vi "Configure Trigger (Video).vi"(0 "VISA resource name":refnum<visa-resource-name>, 1 "Polarity (1: Positive)":u16(ring)=1 items=["Negative", "Positive", "Normal", "Inverted"], 2 "Holdoff Fields (0)":dbl, 5 "Trigger Source (0: Channel 1)":u16(ring) items=["Channel 1"=0, "Channel 2"=1, "Channel 3"=2, "Channel 4"=3, "Digital Channel 0"=14, "Digital Channel 1"=15, "Digital Channel 2"=16, "Digital Channel 3"=17, "Digital Channel 4"=18, "Digital Channel 5"=19, "Digital Channel 6"=20, "Digital Channel 7"=21, "Digital Channel 8"=22, "Digital Channel 9"=23, "Digital Channel 10"=24, "Digital Channel 11"=25, "Digital Channel 12"=26, "Digital Channel 13"=27, "Digital Channel 14"=28, "Digital Channel 15"=29], 7 "Signal Format (0: NTSC)":u16(ring) items=["NTSC", "PAL", "SECAM", "HDTV"], 9 "Trigger Event (0: Odd Fields)":u16(ring) items=["Odd Fields", "Even Fields", "All Fields", "All Lines", "Numeric"], 11 "error in (no error)":errorcluster, 12 "HDTV Format (0: HD1080P24)":u16(ring) items=["HD1080P24", "HD720P60", "HD480P60", "HD1080I50", "HD1080P25", "HD1080I60", "HD1080PSF24", "HD576P50", "HD720P30", "HD720P50", "HD875I60", "HD1080P30", "HD1080P50", "HD1080P60"], 13 "Video Trigger Line (1)":dbl=1.0) -> (4 "VISA resource name out":refnum<visa-resource-name>, 15 "error out":errorcluster)   [LabVIEW 2009, in "Tektronix DPO MSO 2000 4000 Series.lvlib"]
doc: "Configures video trigger settings for an oscilloscope."
uses:
  <instrlib>/Tektronix DPO MSO 2000 4000 Series/Tektronix DPO MSO 2000 4000 Series.lvlib
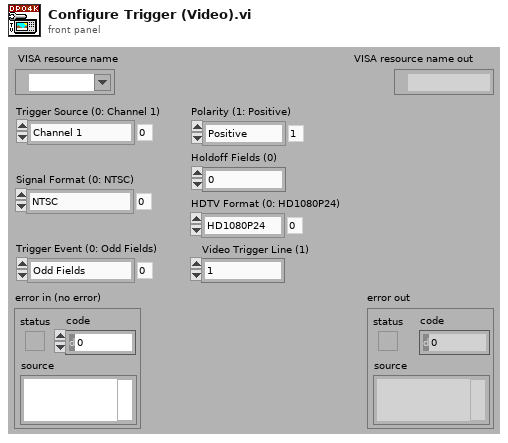
[diagram p1: front panel]
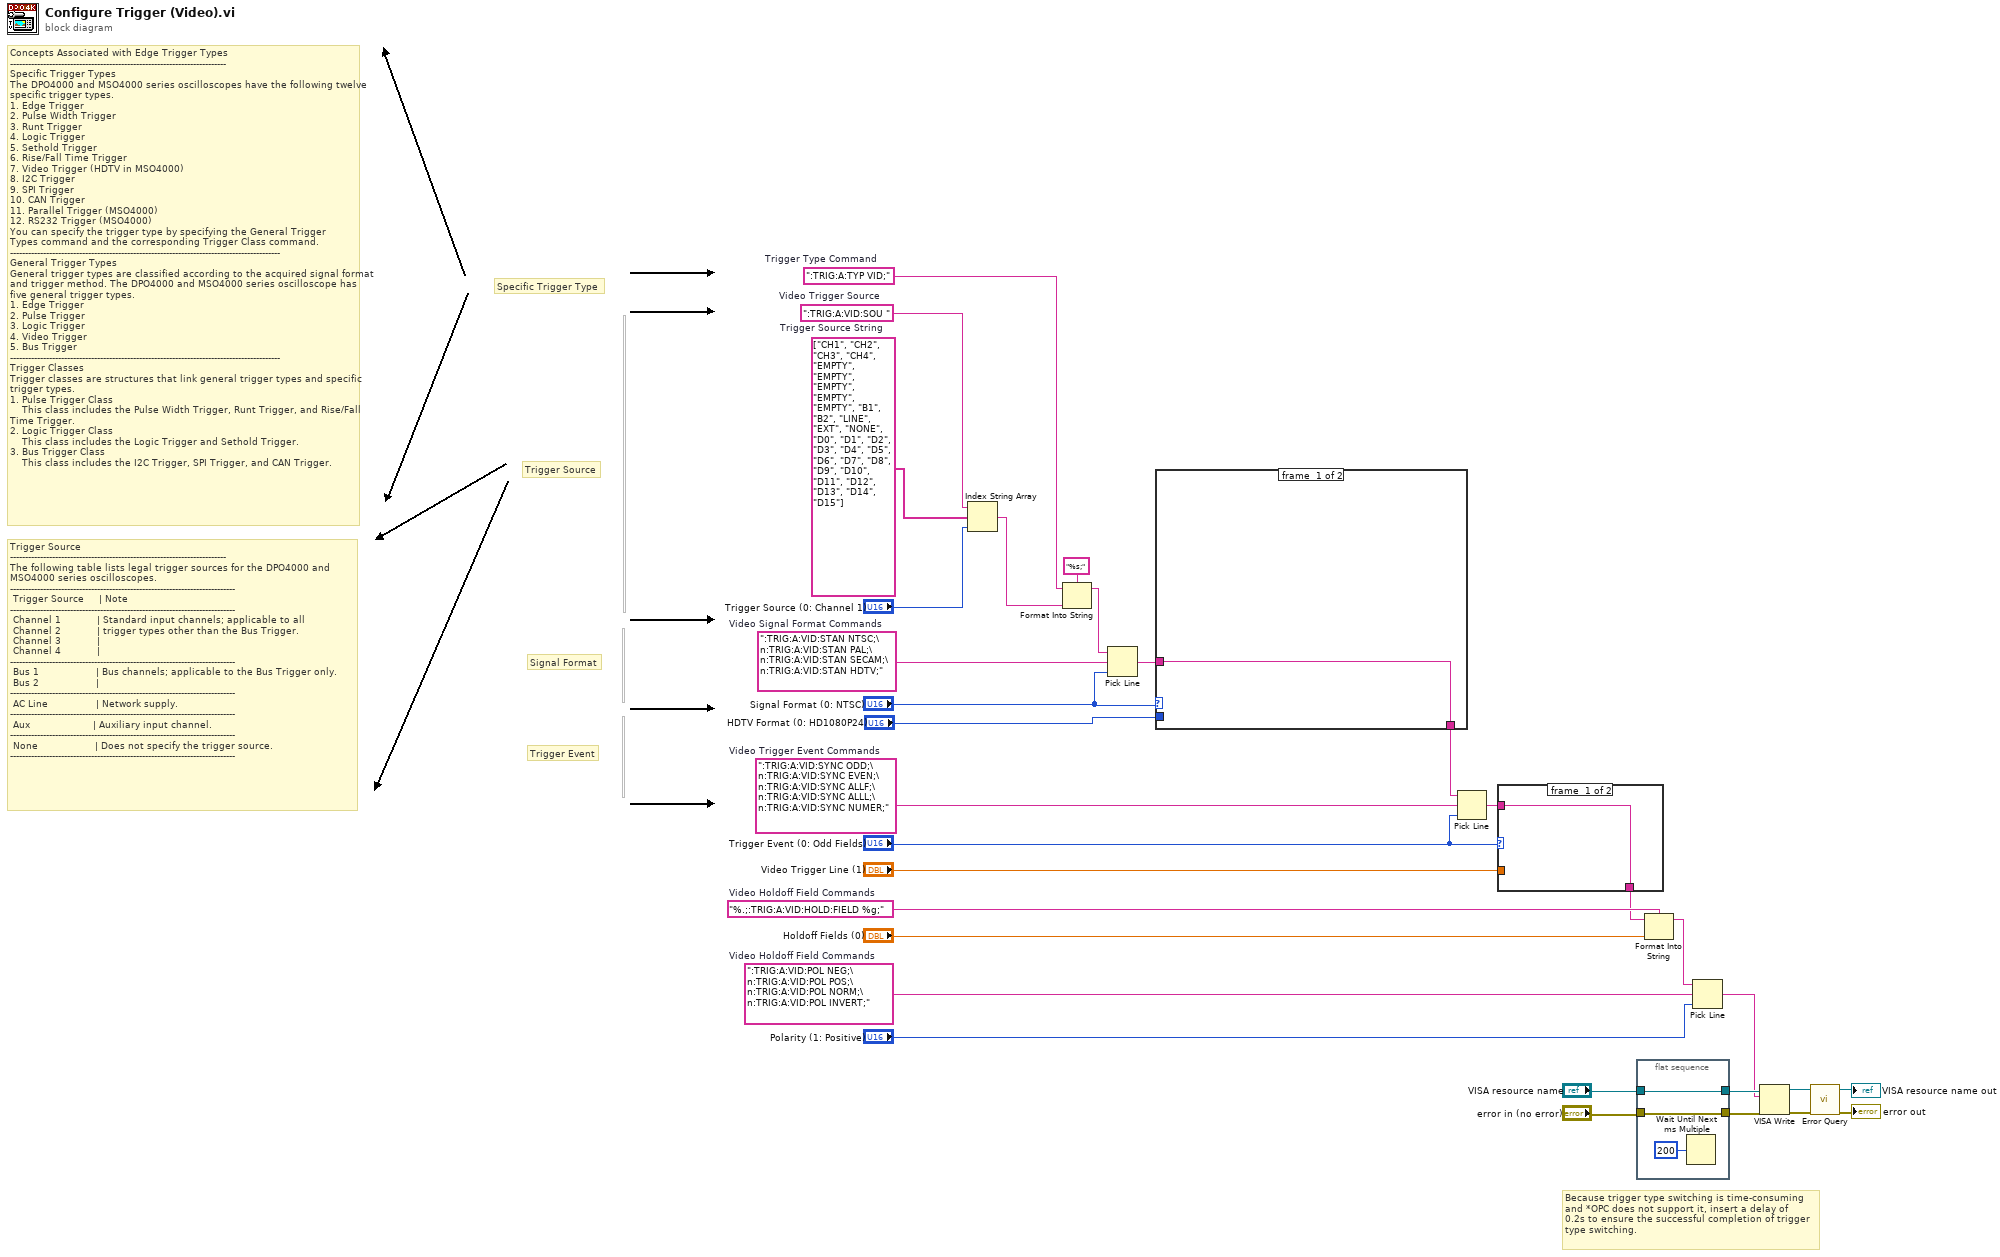
[diagram p0: block diagram]
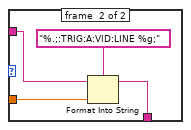
[diagram p2: hidden frame]
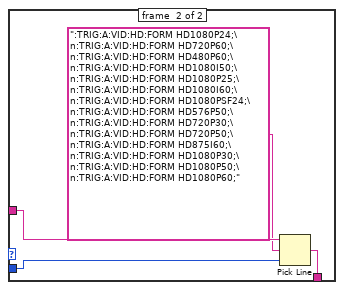
[diagram p3: hidden frame]
diagram:
  w3 = ":TRIG:A:VID:POL NEG;\n:TRIG:A:VID:POL POS;\n:TRIG:A:VID:POL NORM;\n:TRIG:A:VID:POL INVERT;"  # Video Holdoff Field Commands
  w7 = "%.;:TRIG:A:VID:HOLD:FIELD %g;"  # Video Holdoff Field Commands
  w19 = ":TRIG:A:TYP VID;"  # Trigger Type Command
  w20 = string[] ["CH1", "CH2", "CH3", "CH4", "EMPTY", "EMPTY", "EMPTY", "EMPTY", "EMPTY", "B1", "B2", "LINE", "EXT", "NONE", "D0", "D1", "D2", "D3", "D4", "D5", "D6", "D7", "D8", "D9", "D10", "D11", "D12", "D13", "D14", "D15"]  # Trigger Source String
  w22 = ":TRIG:A:VID:SYNC ODD;\n:TRIG:A:VID:SYNC EVEN;\n:TRIG:A:VID:SYNC ALLF;\n:TRIG:A:VID:SYNC ALLL;\n:TRIG:A:VID:SYNC NUMER;"  # Video Trigger Event Commands
  w24 = ":TRIG:A:VID:STAN NTSC;\n:TRIG:A:VID:STAN PAL;\n:TRIG:A:VID:STAN SECAM;\n:TRIG:A:VID:STAN HDTV;"  # Video Signal Format Commands
  w30 = ":TRIG:A:VID:SOU "  # Video Trigger Source
  # "Trigger Source\n------------------------------------------------------------------------\nThe following table lists legal trigger sources for the DPO4000 and MSO4000 series oscilloscopes.\n---------------------------------------------------------------------------\n Trigger Source     | Note                                                           \n---------------------------------------------------------------------------\n Channel 1            | Standard input channels; applicable to all      \n Channel 2            | trigger types other than the Bus Trigger.         \n Channel 3            |     \n Channel 4            |\n---------------------------------------------------------------------------\n Bus 1                   | Bus channels; applicable to the Bus Trigger only.\n Bus 2                   | \n---------------------------------------------------------------------------\n AC Line                | Network supply.\n---------------------------------------------------------------------------\n Aux                     | Auxiliary input channel.\n---------------------------------------------------------------------------\n None                   | Does not specify the trigger source.\n---------------------------------------------------------------------------"
  # "Concepts Associated with Edge Trigger Types\n------------------------------------------------------------------------\nSpecific Trigger Types\nThe DPO4000 and MSO4000 series oscilloscopes have the following twelve specific trigger types.\n1. Edge Trigger\n2. Pulse Width Trigger\n3. Runt Trigger\n4. Logic Trigger\n5. Sethold Trigger\n6. Rise/Fall Time Trigger\n7. Video Trigger (HDTV in MSO4000)\n8. I2C Trigger\n9. SPI Trigger\n10. CAN Trigger\n11. Parallel Trigger (MSO4000)\n12. RS232 Trigger (MSO4000)\nYou can specify the trigger type by specifying the General Trigger \nTypes command and the corresponding Trigger Class command.\n------------------------------------------------------------------------------------------\nGeneral Trigger Types \nGeneral trigger types are classified according to the acquired signal format and trigger method. The DPO4000 and MSO4000 series oscilloscope has five general trigger types.\n1. Edge Trigger\n2. Pulse Trigger\n3. Logic Trigger\n4. Video Trigger\n5. Bus Trigger\n------------------------------------------------------------------------------------------\nTrigger Classes\nTrigger classes are structures that link general trigger types and specific trigger types.\n1. Pulse Trigger Class\n    This class includes the Pulse Width Trigger, Runt Trigger, and Rise/Fall Time Trigger.\n2. Logic Trigger Class\n    This class includes the Logic Trigger and Sethold Trigger.\n3. Bus Trigger Class\n    This class includes the I2C Trigger, SPI Trigger, and CAN Trigger."
  # "Because trigger type switching is time-consuming\nand *OPC does not support it, insert a delay of\n0.2s to ensure the successful completion of trigger\ntype switching."
  # "Trigger Event"
  # "Signal Format"
  # "Trigger Source"
  # "Specific Trigger Type"
  n1 = Index String Array(1:"Trigger Source (0: Channel 1)", 2:w20, 3:w30) -> (0:w23:string)
  n2 = Format Into String(format string="%s;", initial string=w19, w23) -> (resulting string=w21:string)  [unwired: 1 in, 1 out]
  n3 = Pick Line(string ("")=w21, multi-line string=w24, line index="Signal Format (0: NTSC)") -> (output string=w13:string)
  n4 = case shown="0, Default" "Signal Format (0: NTSC)" {
    tunnel: w13 -> [w32 w36]
    tunnel: "HDTV Format (0: HD1080P24)" -> [_ w34]
    tunnel: [w32 w33] -> w11
    frame #0 {
    }
    frame #1 {
      n5 = Pick Line(string ("")=w36, multi-line string=":TRIG:A:VID:HD:FORM HD1080P24;\n:TRIG:A:VID:HD:FORM HD720P60;\n:TRIG:A:VID:HD:FORM HD480P60;\n:TRIG:A:VID:HD:FORM HD1080I50;\n:TRIG:A:VID:HD:FORM HD1080P25;\n:TRIG:A:VID:HD:FORM HD1080I60;\n:TRIG:A:VID:HD:FORM HD1080PSF24;\n:TRIG:A:VID:HD:FORM HD576P50;\n:TRIG:A:VID:HD:FORM HD720P30;\n:TRIG:A:VID:HD:FORM HD720P50;\n:TRIG:A:VID:HD:FORM HD875I60;\n:TRIG:A:VID:HD:FORM HD1080P30;\n:TRIG:A:VID:HD:FORM HD1080P50;\n:TRIG:A:VID:HD:FORM HD1080P60;", line index=w34) -> (output string=w33:string)
    }
  }
  n6 = Pick Line(string ("")=w11, multi-line string=w22, line index="Trigger Event (0: Odd Fields)") -> (output string=w9:string)
  n7 = case shown="0..3, Default" "Trigger Event (0: Odd Fields)" {
    tunnel: w9 -> [w37 w40]
    tunnel: [w37 w38] -> w6
    tunnel: "Video Trigger Line (1)" -> [_ w41]
    frame #0 {
    }
    frame #1 {
      n8 = Format Into String(format string="%.;:TRIG:A:VID:LINE %g;", initial string=w40, w41) -> (resulting string=w38:string)  [unwired: 1 in, 1 out]
    }
  }
  n9 = flat-sequence {
    tunnel: "VISA resource name" -> [w43]
    tunnel: [w43] -> w18
    tunnel: "error in (no error)" -> [w42]
    tunnel: [w42] -> w17
    frame #0 {
      n10 = Wait Until Next ms Multiple(millisecond multiple=u32 200) -> ()  [unwired: 1 out]
    }
  }
  n11 = Format Into String(format string=w7, initial string=w6, "Holdoff Fields (0)") -> (resulting string=w4:string)  [unwired: 1 in, 1 out]
  n12 = Pick Line(string ("")=w4, multi-line string=w3, line index="Polarity (1: Positive)") -> (output string=w1:string)
  n13 = VISA Write(VISA resource name=w18, write buffer=w1, error in (no error)=w17) -> (VISA resource name out=w29:refnum<visa-resource-name>, error out=w28:errorcluster)  [unwired: 1 out]
  n14 = call <instrlib>:"Error Query.vi"("error in (no error)"=w28, "VISA resource name"=w29) -> ("error out"=→"error out":errorcluster, "VISA resource name out"=→"VISA resource name out":refnum<visa-resource-name>)  [unwired: 6 in, 2 out]
